vi "is container class.vi"(8 "error in":errorcluster, 11 "module editor node in":refnum<class "module editor node.lvclass">) -> (0 "error out":errorcluster, 2 "container?":bool, 3 "module editor node out":refnum<class "module editor node.lvclass">)   [LabVIEW 2013, in "PL Framework Configuration Tool.lvlib" / "module editor node.lvclass"]
uses:
  module editor node.lvclass
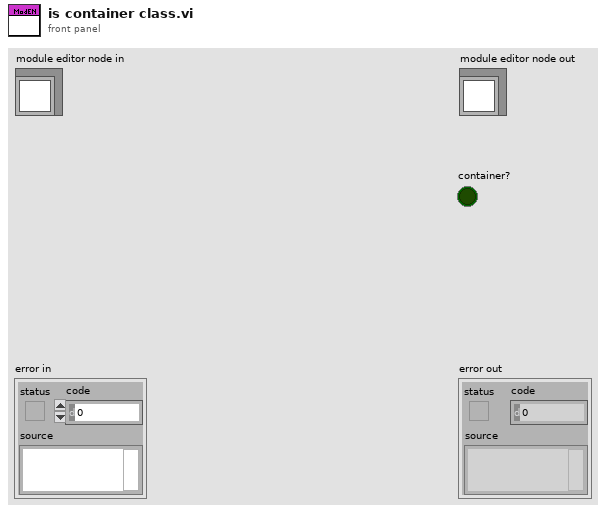
[diagram p1: front panel]
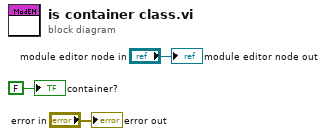
[diagram p0: block diagram]
diagram:
  "error out" <- "error in"
  "module editor node out" <- "module editor node in"
  "container?" <- FALSE ("container?")
